vi "beginStopPlayVSS.vi"(8 "error in (no error)":errorcluster, 10 "Game in":refnum<class "Game.lvclass">, 11 "StopPlayVSS in":refnum<class "StopPlayVSS.lvclass">) -> (0 "error out":errorcluster, 2 "Boolean":bool, 3 "StopPlayVSS out":refnum<class "StopPlayVSS.lvclass">)   [LabVIEW 2020, in "StopPlayVSS.lvclass"]
uses:
  StopPlayVSS.lvclass
  Game_class/Game.lvclass
  Game_class/Game.lvclass/Game.ctl
  Game_class/Read Referee.vi
  Referee_class/Referee.lvclass
panel:
  in  "queue":T1(array[ring])
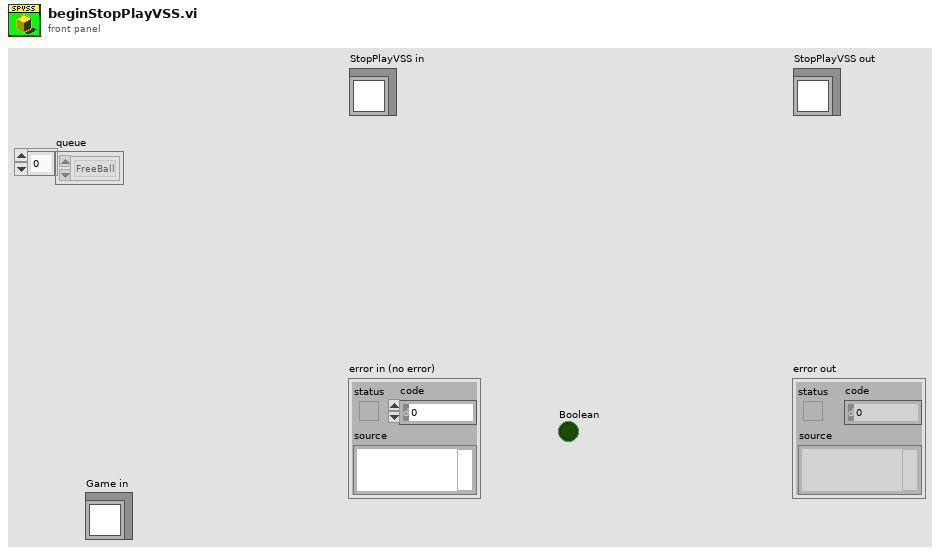
[diagram p1: front panel]
types:
  T1 = enum16{"FreeBall", "PrepareFreeBall", "GoalKickEnemy", "GoalKickAlly", "KickoffAlly", "KickoffEnemy", "PrepareGoalKickEnemy", "PrepareGoalKickAlly", "Stop", "PrepareKickoffEnemy", "PrepareKickoffAlly", "PreparePenaltyEnemy", "Timeout", "DeadBall", "NormalGame", "KickPenaltyAlly", "PenaltyEnemy", "BallChallenge", "PreparePenaltyAlly", "Halt"}[]
  T2 = enum16{"AUTO", "GAME_ON", "STOP", "KICKOFF", "FREE_BALL", "GOAL_KICK", "PENALTY_KICK", "FREE_KICK"}
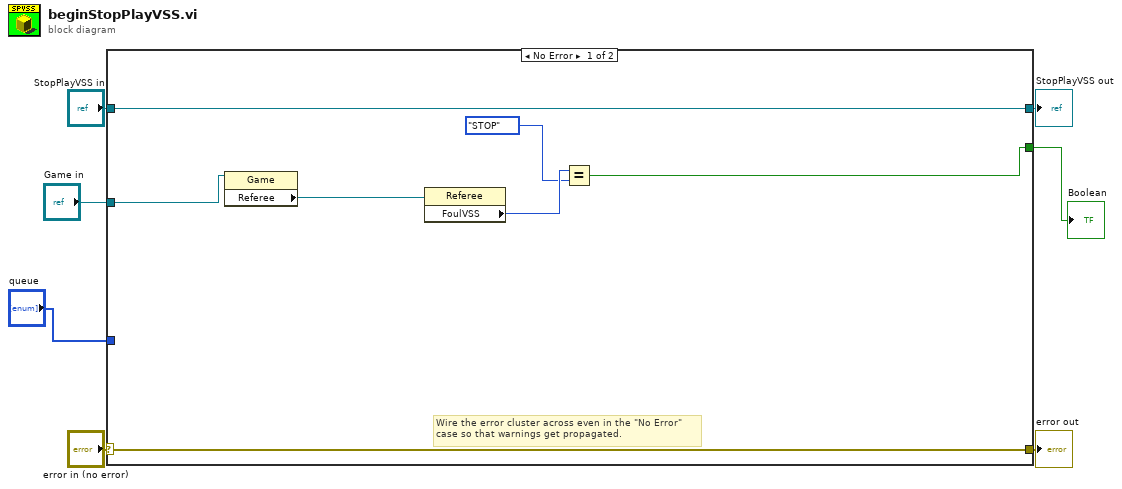
[diagram p0: block diagram]
diagram:
  n1 = case shown="No Error" "error in (no error)" {
    selector: "error in (no error)" -> [w13 w16]
    tunnel: [w13 w16] -> w6
    tunnel: [w14 w15] -> w4
    tunnel: "StopPlayVSS in" -> [w14 w15]
    tunnel: "Game in" -> [w9 _]
    tunnel: [w8 _] -> w2
    tunnel: "queue" -> [_ _]
    frame No Error {
      # "Wire the error cluster across even in the \"No Error\"\ncase so that warnings get propagated."
      n2 = property class="Game"(reference=w9) -> ("Referee"=w12:refnum<class "Referee.lvclass">)  [unwired: 1 in, 2 out]
      n3 = property class="Referee"(reference=w12) -> ("FoulVSS"=w11:T2)  [unwired: 1 in, 2 out]
      n4 = Equal?(x=w11, y=T2."STOP" ("FoulVSS")) -> (x = y?=w8:bool)
    }
    frame Error {
    }
  }
  "error out" <- w6
  "StopPlayVSS out" <- w4
  "Boolean" <- w2
